vi "SERIAL_StopLoop.vi"(0 "Stop?":bool, 1 "Update?":bool) -> (2 "Stop?":bool)   [LabVIEW 2014]
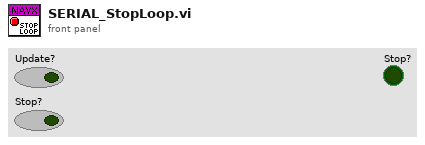
[diagram p1: front panel]
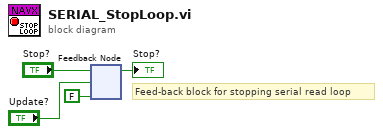
[diagram p0: block diagram]
diagram:
  # "Feed-back block for stopping serial read loop"
  n1 = feedback-in #1("Stop?", "Update?") -> ()
  n2 = feedback #1(FALSE ("Stop?")) -> (→"Stop?":bool)
